vi "Actor Core.vi"(8 "error in":errorcluster, 11 "Launch View in":refnum<class "Launch View.lvclass">) -> (0 "error out":errorcluster, 3 "Actor out":refnum<class "Actor.lvclass">)   [LabVIEW 2020, in "Launch View.lvlib" / "Launch View.lvclass"]
doc: "(<B>Filename</B>: Actor Framework.lvlib:Actor.lvclass:Actor Core.vi)\n\nReceives messages to the actor, reacts to them, and initiates any error handling that may shut the actor down.\n\nDescendant classes may override this VI to append parallel tasks for the actor to complete while it handles messages. Overrides use the Call Parent Method node."
uses:
  Launch View.lvclass
  <vilib>/ActorFramework/Actor/Actor.lvclass
  Launch View.lvclass/Launch View.ctl
  <vilib>/ActorFrameworkMVC/Abstract View/Abstract View/Abstract View.lvclass
panel:
  out "Information":string="Initializing..."
  # "copyright(c) 2015-2017 tmirob inc. all rights reserved"
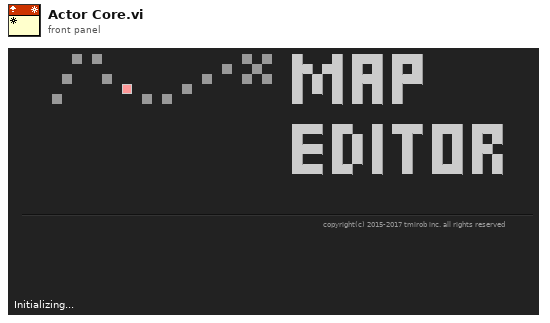
[diagram p1: front panel]
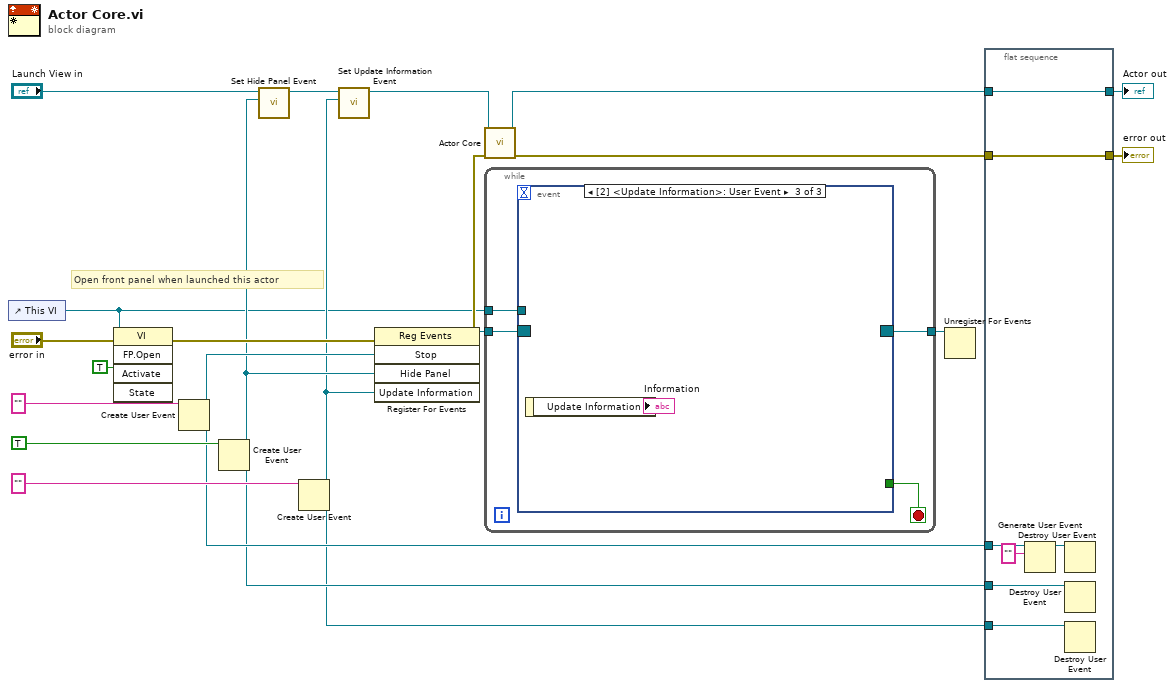
[diagram p0: block diagram]
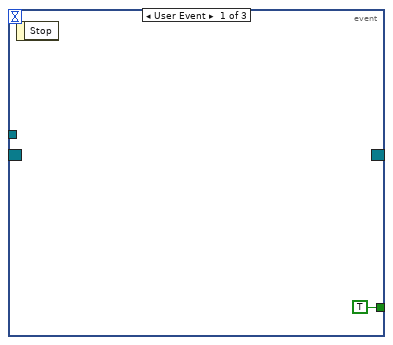
[diagram p2: hidden frame]
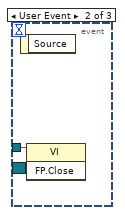
[diagram p3: hidden frame]
diagram:
  # "Open front panel when launched this actor"
  n1 = control-ref of="This VI"() -> (w1:refnum<vi>)
  n2 = invoke class="VI" method="FP.Open"(reference=w1, error in="error in", "Activate"=TRUE ("Activate?")) -> (error out=w5:errorcluster)  [unwired: 2 in, 4 out]
  n3 = Create User Event(user event datatype="" ("Stop")) -> (user event=w15:refnum<user-event>)  [unwired: 1 in, 1 out]
  n4 = Create User Event(user event datatype=TRUE ("Hide Panel")) -> (user event=w3:refnum<user-event>)  [unwired: 1 in, 1 out]
  n5 = call "Set Hide Panel Event.vi"("Hide Panel Event"=w3, "Launch View in"="Launch View in") -> ("Launch View out"=w7:refnum<class "Launch View.lvclass">)  [unwired: 9 in]
  n6 = Create User Event(user event datatype="" ("Update Information")) -> (user event=w2:refnum<user-event>)  [unwired: 1 in, 1 out]
  n7 = call "Set Update Information Event.vi"("Update Information Event"=w2, "Launch View in"=w7) -> ("Launch View out"=w6:refnum<class "Launch View.lvclass">)  [unwired: 9 in]
  n8 = register-events(error in=w5, w15, w3, w2) -> (reference out=w20:refnum<event-registration>, error out=w12:errorcluster)  [unwired: 1 in]
  n9 = call-parent "Actor Core.vi"("error in"=w12, "Abstract View in"=w6) -> ("error out"=w13:errorcluster, "Actor out"=w14:refnum<class "Actor.lvclass">)  [unwired: 8 in]
  n10 = while {
    tunnel: w20 -> [w24]
    tunnel: [w23] -> w19
    tunnel: w1 -> [w21]
    stop <- w22 stop-if-true
    n11 = event shown="[2] <Update Information>: User Event" {
      selector: w24 -> [_ _ _]
      dyn-events: [_ _ _] -> w23
      timeout: _ -> [_ _ _]
      tunnel: [TRUE _ _] -> w22
      tunnel: w21 -> [_ w26 _]
      event User Event {
        n12 = event-data() -> ()  [unwired: 1 in, 1 out]
      }
      event User Event {
        n13 = event-data() -> ()  [unwired: 1 in, 1 out]
        n14 = invoke class="VI" method="FP.Close"(reference=w26) -> ()  [unwired: 2 in, 3 out]
      }
      event User Event {
        n15 = event-data() -> ("Update Information"=→"Information":string)  [unwired: 1 in]
      }
    }
  }
  n16 = Unregister For Events(event registration refnum=w19) -> ()  [unwired: 1 in, 1 out]
  n17 = flat-sequence {
    tunnel: w15 -> [w33]
    tunnel: w3 -> [w31]
    tunnel: w2 -> [w30]
    tunnel: w14 -> [w29]
    tunnel: [w29] -> w11
    tunnel: [w28] -> w10
    tunnel: w13 -> [w28]
    frame #0 {
      n18 = Generate User Event(user event=w33, event data cluster="" ("event data")) -> (user event out=w34:refnum<user-event>)  [unwired: 2 in, 1 out]
      n19 = Destroy User Event(user event=w34) -> ()  [unwired: 1 in, 1 out]
      n20 = Destroy User Event(user event=w31) -> ()  [unwired: 1 in, 1 out]
      n21 = Destroy User Event(user event=w30) -> ()  [unwired: 1 in, 1 out]
    }
  }
  "error out" <- w10
  "Actor out" <- w11
